vi "Set Enabled Cameras.vi"(8 "error in (no error)":errorcluster, 10 "Cameras Enabled":bool[](array[boolean]), 11 "Hamamatsu Camera in":refnum<class "Hamamatsu Camera.lvclass">) -> (0 "error out":errorcluster, 3 "Hamamatsu Camera out":refnum<class "Hamamatsu Camera.lvclass">)   [LabVIEW 2018, in "Hamamatsu Camera.lvlib" / "Hamamatsu Camera.lvclass"]
uses:
  Hamamatsu Camera.lvclass
  Hamamatsu Camera.lvclass/Hamamatsu Camera.ctl
  Resources/GLOBAL/GLOBAL Time-critical.vi
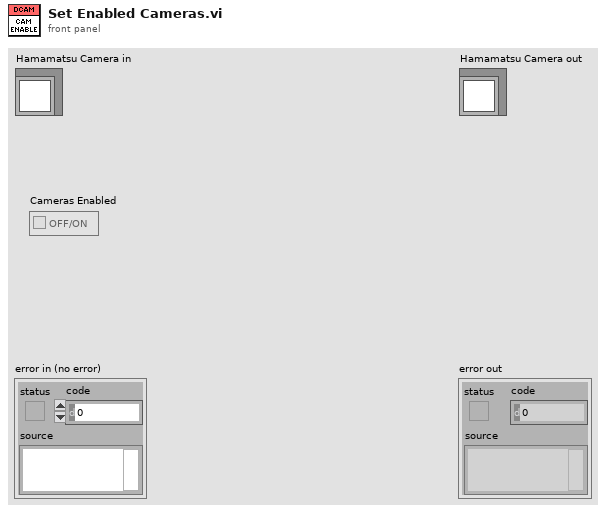
[diagram p1: front panel]
types:
  T1 = typedef "Physical Camera Assignment.ctl" = cluster{"Channel Name":string, "Camera Type":T2, "Serial Number":string, "Flip Vertically":bool, "Flip Horizontally":bool, "photonsPerCount":dbl, "wavelength":i16}
  T2 = typedef "Camera Type.ctl" = enum16{"Hamamatsu"}
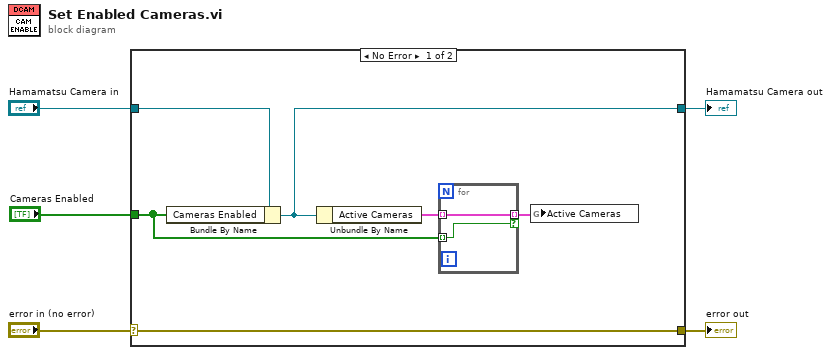
[diagram p0: block diagram]
diagram:
  n1 = case shown="No Error" "error in (no error)" {
    selector: "error in (no error)" -> [w11 w15]
    tunnel: [w11 w15] -> w4
    tunnel: [w9 w14] -> w2
    tunnel: "Hamamatsu Camera in" -> [w10 w14]
    tunnel: "Cameras Enabled" -> [w6 _]
    frame No Error {
      n2 = Bundle By Name(cluster=w10, "Cameras Enabled"=w6) -> (w9:refnum<class "Hamamatsu Camera.lvclass">)
      n3 = Unbundle By Name(w9) -> ("Active Cameras"=w8:T1[])
      n4 = for {
        tunnel: w8 -> [w13] mode=indexing
        tunnel: [w13] -> w7 mode=indexing if=w12
        tunnel: w6 -> [w12] mode=indexing
      }
      n5 = global write "GLOBAL Time-critical.vi" "Active Cameras"(w7) -> ()
    }
    frame Error {
    }
  }
  "error out" <- w4
  "Hamamatsu Camera out" <- w2
